vi "FileTransferTarget2Host.vi"() -> ()   [LabVIEW 2010]
uses:
  <vilib>/FTP/NI_FTP.lvlib
panel:
  out "error out":errorcluster
  out "file error":errorcluster
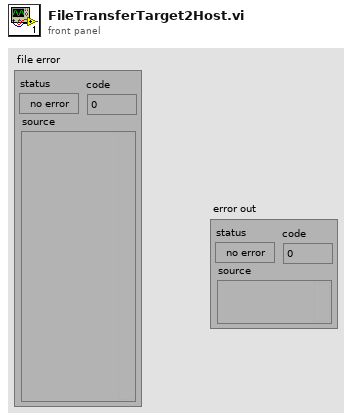
[diagram p1: front panel]
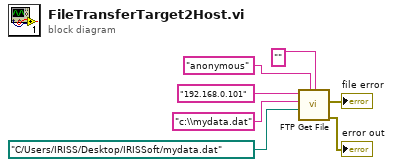
[diagram p0: block diagram]
diagram:
  n1 = call <vilib>:"FTP Get File.vi"("password"="", "user"="anonymous", "local path"=path "C:/Users/IRISS/Desktop/IRISSoft/mydata.dat", "remote path"="c:\\mydata.dat", "host"="192.168.0.101") -> ("error out"=→"error out":errorcluster, "file error"=→"file error":errorcluster)  [unwired: 5 in]
